vi "tool.vi"() -> ()   [LabVIEW 2020]
uses:
  <vilib>/Waveform/WDTFileIO.llb/ Write Waveforms to File (1D).vi
  <vilib>/Waveform/WDTFileIO.llb/Export Waveforms To Spreadsheet File (1D).vi
panel:
  out "从文件读取的波形":waveform(dbl)[](graph)
  out "写入文件的波形":waveform(dbl)[](graph)
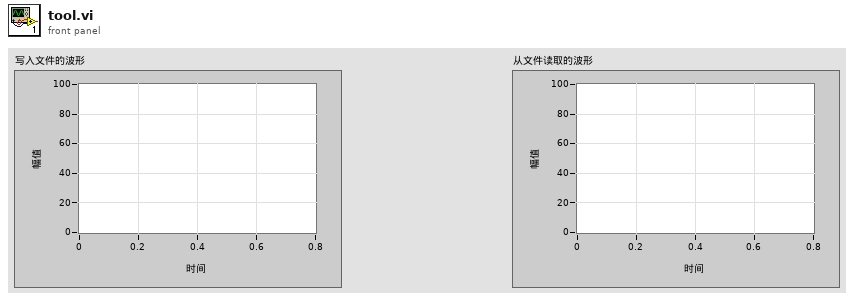
[diagram p1: front panel]
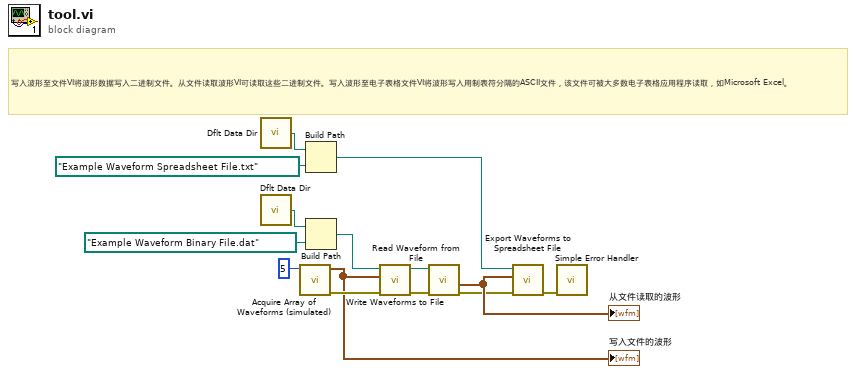
[diagram p0: block diagram]
diagram:
  # "写入波形至文件VI将波形数据写入二进制文件。从文件读取波形VI可读取这些二进制文件。写入波形至电子表格文件VI将波形写入用制表符分隔的ASCII文件，该文件可被大多数电子表格应用程序读取，如Microsoft Excel。"
  n1 = call <vilib>:"Dflt Data Dir.vi"() -> ("App:Default Data Directory"=w7:path)
  n2 = call <vilib>:"Dflt Data Dir.vi"() -> ("App:Default Data Directory"=w4:path)
  n3 = call "Acquire Array of Waveforms (simulated).vi"("创建的波形数量"=5 ("# of waveforms to create")) -> ("error out"=w9:cluster{"状态":bool, "代码":i32, "源":string}, "波形数组"=w1:waveform(dbl)[])  [unwired: 9 in]
  "写入文件的波形" <- w1
  n4 = Build Path(base path=w7, name or relative path=path "Example Waveform Spreadsheet File.txt" ("default name")) -> (appended path=w3:path)
  n5 = Build Path(base path=w4, name or relative path=path "Example Waveform Binary File.dat" ("default name")) -> (appended path=w2:path)
  n6 = call-poly <vilib>:"Write Waveforms to File.vi"("error in (no error)"=w9, "waveform array"=w1, "file path (dialog if empty)"=w2) -> ("error out"=w11:errorcluster, "new file path (Not A Path if cancelled)"=w13:path)  [unwired: 7 in]
  n7 = call <vilib>:"Read Waveform from File.vi"("error in (no error)"=w11, "file path (dialog if empty)"=w13) -> ("error out"=w10:errorcluster, "all waveforms in record"=w12:waveform(dbl)[])  [unwired: 4 in, 2 out]
  "从文件读取的波形" <- w12
  n8 = call-poly <vilib>:"Export Waveforms to Spreadsheet File.vi"("error in (no error)"=w10, "waveforms"=w12, "file path (dialog if empty)"=w3) -> ("error out"=w8:errorcluster)  [unwired: 7 in, 1 out]
  n9 = call <vilib>:"Simple Error Handler.vi"("error in (no error)"=w8) -> ()  [unwired: 4 in, 5 out]
